vi "load_loads.vi"(9 "Nodes":string[](array[string]), 10 "Events":string[](array[string]), 11 "Diretório de trabalho":path=path "C:/ATP/ATPDraw/Projects_Flavio") -> (2 "Loads (out)":string[](array[string]))   [LabVIEW 2020]
uses:
  <vilib>/Utility/file.llb/Read Delimited Spreadsheet (string).vi
panel:
  in  "Lista de condições (arquivo.txt) 3":string="list_X.txt"
  in  "Lista de condições (arquivo.txt) 2":string="list_GDs.txt"
  in  "Lista de condições (arquivo.txt)":string="list_all_loads.txt"
  # "SELECIONA NÓS"
  # "quando N = ALL"
  # "ENTRADAS"
  # "CONSTANTES"
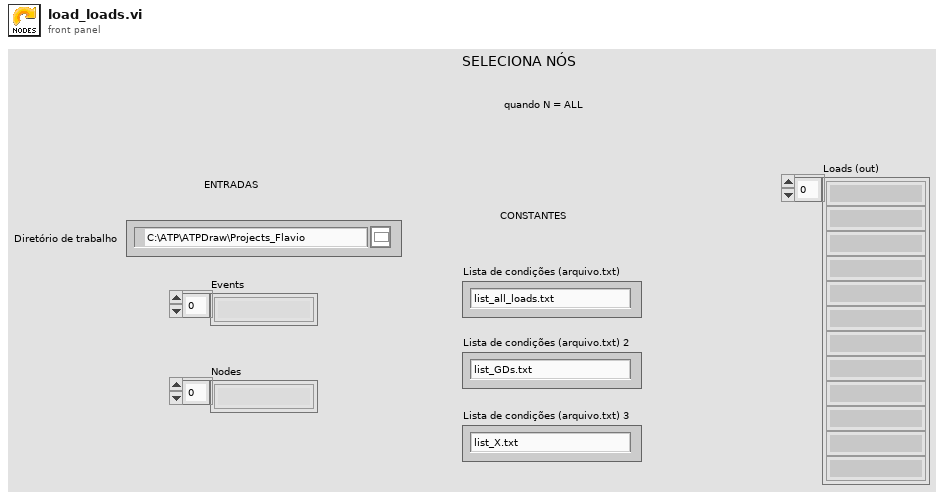
[diagram p1: front panel]
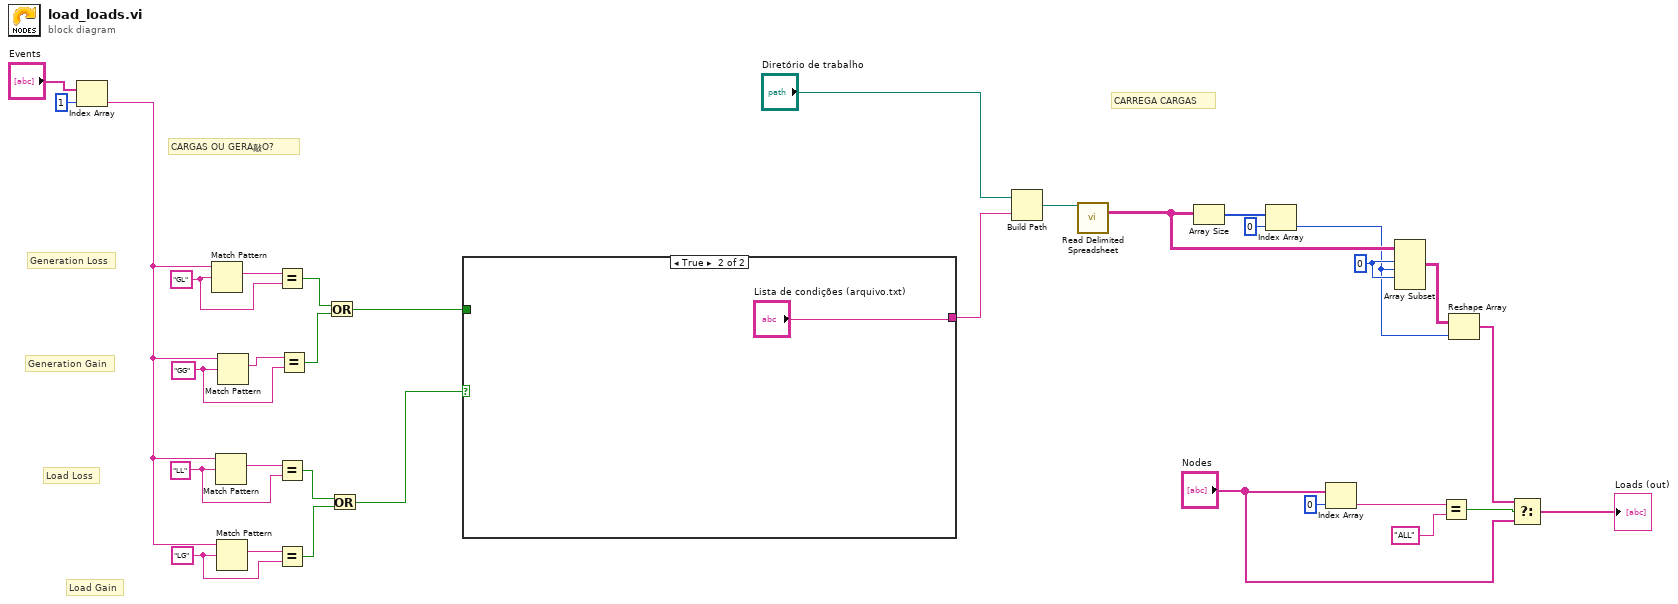
[diagram p0: block diagram]
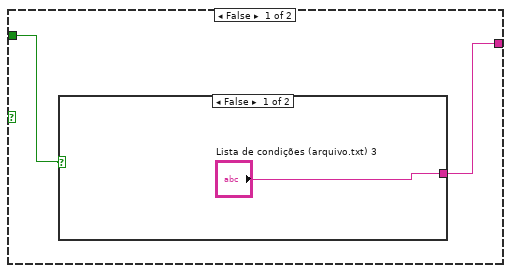
[diagram p2: hidden frame]
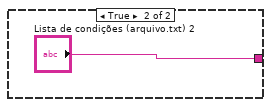
[diagram p3: hidden frame]
diagram:
  w15 = "GG" ("regular expression")
  w12 = "GL" ("regular expression")
  w13 = "LL" ("regular expression")
  w14 = "LG" ("regular expression")
  w27 = 0 ("index")
  # "CARGAS OU GERA敲O?"
  # "Generation Gain"
  # "Generation Loss"
  # "Load Gain"
  # "Load Loss"
  # "CARREGA CARGAS"
  n1 = Index Array(array="Events", index=1) -> (element=w6:string)
  n2 = Match Pattern(string=w6, regular expression=w12) -> (match substring=w16:string)  [unwired: 1 in, 3 out]
  n3 = Match Pattern(string=w6, regular expression=w13) -> (match substring=w11:string)  [unwired: 1 in, 3 out]
  n4 = Match Pattern(string=w6, regular expression=w14) -> (match substring=w18:string)  [unwired: 1 in, 3 out]
  n5 = Match Pattern(string=w6, regular expression=w15) -> (match substring=w10:string)  [unwired: 1 in, 3 out]
  n6 = Equal?(x=w16, y=w12) -> (x = y?=w17:bool)
  n7 = Equal?(x=w11, y=w13) -> (x = y?=w5:bool)
  n8 = Equal?(x=w18, y=w14) -> (x = y?=w4:bool)
  n9 = Equal?(x=w10, y=w15) -> (x = y?=w7:bool)
  n10 = Or(x=w17, y=w7) -> (x .or. y?=w1:bool)
  n11 = Or(x=w5, y=w4) -> (x .or. y?=w2:bool)
  n12 = case shown="True" w2 {
    tunnel: [w35 "Lista de condições (arquivo.txt)"] -> w3
    tunnel: w1 -> [w34 _]
    frame False {
      n13 = case shown="False" w34 {
        tunnel: ["Lista de condições (arquivo.txt) 3" "Lista de condições (arquivo.txt) 2"] -> w35
        frame False {
        }
        frame True {
        }
      }
    }
    frame True {
    }
  }
  n14 = Build Path(base path="Diretório de trabalho", name or relative path=w3) -> (appended path=w29:path)
  n15 = call-poly <vilib>:"Read Delimited Spreadsheet.vi"("file path (dialog if empty)"=w29) -> ("all rows"=w26:string[][])  [unwired: 9 in, 5 out]
  n16 = Array Size(array=w26) -> (size(s)=w25:i32[])
  n17 = Index Array(array=w25, index=0) -> (element=w21:i32)
  n18 = Index Array(array="Nodes", index=0) -> (element=w32:string)
  n19 = Array Subset(array=w26, index (row)=w27, length (row)=w21, index (col)=w27) -> (w22:string[][])  [unwired: 1 in]
  n20 = Equal?(x=w32, y="ALL") -> (x = y?=w30:bool)
  n21 = Reshape Array(w22, w21) -> (w20:string[])
  n22 = Select(t=w20, s=w30, f="Nodes") -> (s? t:f=→"Loads (out)":string[])
